vi "qCTV.vi"(0 "System no.":i32=1 min=1 max=4 step=1, 2 "Axes to query":string[](array[string]), 3 "All axes?":bool, 4 "Axis identifier?":bool=TRUE, 5 "error in":errorcluster) -> (14 "Target values":dbl[](array[numeric]) format="%.6f", 19 "error out":errorcluster)   [LabVIEW 2020]
doc: "Returns the last valid target value (in physical units) for the currently selected control mode.\n\nC-413: If All axes? = TRUE, then Axis identifier? can be FALSE."
panel:
  # "Returns last valid target value for currently selected control mode."
  # "If all axes: use"
  # "Query"
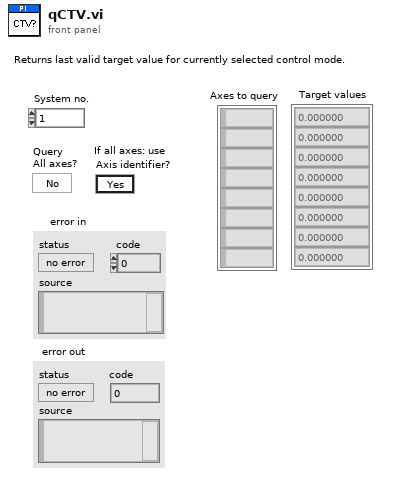
[diagram p1: front panel]
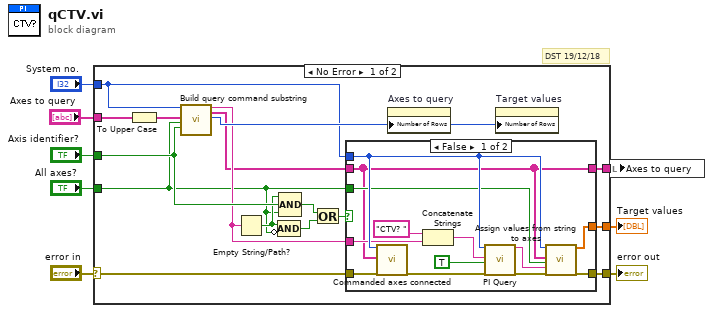
[diagram p0: block diagram]
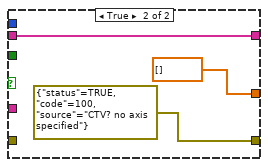
[diagram p2: hidden frame]
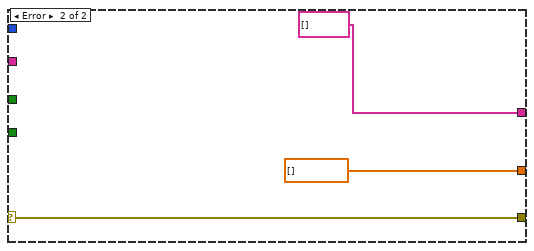
[diagram p3: hidden frame]
diagram:
  # "DST 19/12/18"
  n1 = case shown="No Error" "error in" {
    selector: "error in" -> [w13 w41]
    tunnel: [w24 dbl[] [] ("Values")] -> w8
    tunnel: "Axes to query" -> [w23 _]
    tunnel: [w16 w41] -> w6
    tunnel: "System no." -> [w20 _]
    tunnel: [w10 string[] [] ("Axes to query out")] -> w4
    tunnel: "Axis identifier?" -> [w18 _]
    tunnel: "All axes?" -> [w9 _]
    frame No Error {
      n2 = To Upper Case(1:w23) -> (0:w22:string[])
      n3 = call "Build query command substring.vi"("System no."=w20, "Axes to query in"=w22, "Query\nAll axes?"=w9, "For all axes: use\nAxis identifier?"=w18) -> ("Command substring"=w15:string, "Axes to query out"=w11:string[], "Number of rows"=w21:u32)  [unwired: 2 in, 11 out]
      n4 = Empty String/Path?(string/path=w15) -> (empty?=w14:bool)
      n5 = Compound Arithmetic op=AND(w14, invert w9) -> (w19:bool)
      n6 = Compound Arithmetic op=AND(w14, w18, w9) -> (w17:bool)
      n7 = Or(x=w17, y=w19) -> (x .or. y?=w12:bool)
      n8 = case shown="False" w12 {
        tunnel: [w34 dbl[] [] ("Values")] -> w24
        tunnel: w20 -> [w33 _]
        tunnel: w11 -> [w25 w38]
        tunnel: w9 -> [w32 _]
        tunnel: [w30 errorcluster {"status"=TRUE, "code"=100, "source"="CTV? no axis specified"} ("error out")] -> w16
        tunnel: w15 -> [w29 _]
        tunnel: w13 -> [w28 _]
        tunnel: [w25 w38] -> w10
        frame False {
          n9 = call "Commanded axes connected.vi"("System no."=w33, "Commanded axes"=w25, "error in"=w28) -> ("error out"=w31:errorcluster)  [unwired: 1 in, 15 out]
          n10 = Concatenate Strings("CTV? ", w29) -> (w35:string)
          n11 = call "PI Query.vi"("System no."=w33, "String to send"=w35, "Attach termination char.?"=TRUE ("Attach Linefeed?"), "error in"=w31) -> ("String read"=w27:string, "error out"=w26:errorcluster)  [unwired: 3 in, 11 out]
          n12 = call "Assign values from string to axes.vi"("System no."=w33, "Queried axes"=w25, "All axes queried?"=w32, "Input String"=w27, "error in"=w26) -> ("Values"=w34:dbl[], "error out"=w30:errorcluster)  [unwired: 4 in, 9 out]
        }
        frame True {
        }
      }
      n13 = property on="Axes to query" class="Arr (strict)"("Number of Rows"=w21) -> ()  [unwired: 2 in, 2 out]
      n14 = property on="Target values" class="Arr (strict)"("Number of Rows"=w21) -> ()  [unwired: 2 in, 2 out]
    }
    frame Error {
    }
  }
  "error out" <- w6
  "Target values" <- w8
  n15 = local write "Axes to query"(w4) -> ()
